vi "Pinholes.vi"(4 "Current Threshold [nA]":dbl, 5 "settling\ndelay":i32) -> (1 "excluded channels":i32[](array[numeric]), 2 "Current [nA]":dbl[](array[numeric]), 3 "Flag":i32[](array[numeric]))   [LabVIEW 2018]
uses:
  general_VIs/globals/QC_MeasurementSetup.vi
  InstrControl/Switching/Switching.lvclass
  InstrControl/SupplyControl/SupplyControl.lvclass
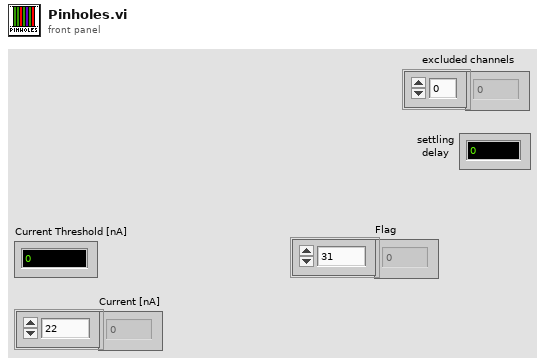
[diagram p1: front panel]
types:
  T1 = cluster{"Bias Supply":refnum<class "SupplyControl.lvclass">, "SMU":refnum<class "SupplyControl.lvclass">, "LCR":refnum<class "LCRControl.lvclass">, "ProbeStation":refnum<class "ProbeStationControl.lvclass">, "Arduino":refnum<class "ArduinoControl.lvclass">, "Measurement switch":refnum<class "Switching.lvclass">, "Probe Card Channels":i32, "Bias Voltage [V]":dbl, "First strip":i32, "Last strip":i32, "Base Voltage [V]":dbl, "Base Ramp Step [V]":dbl, "Base Ramp Interval [ms]":u32, "High Voltage [V]":dbl, "High Ramp Step [V]":dbl, "High Ramp Interval [ms]":u32, "AC frequency [Hz]":i32, "AC amplitude [V]":dbl, "RC Configuration":u16, "Single Needle":bool, "Temperature Readout":enum16{"Read Arduino", "Enter manually"}, "Fraction of good strips [%]":dbl, "Measurement switch used?":bool, "Matrix X Channels":cluster{"Mux1 C1":i32, "Mux1 C2":i32, "Mux2 C1":i32, "Mux2 C2":i32}, "Pinholes Y/N":bool, "Capacitance Y/N":bool, "Resistance Y/N":bool, "Bias Supply Name":string, "SMU Name":string, "LCR Name":string}
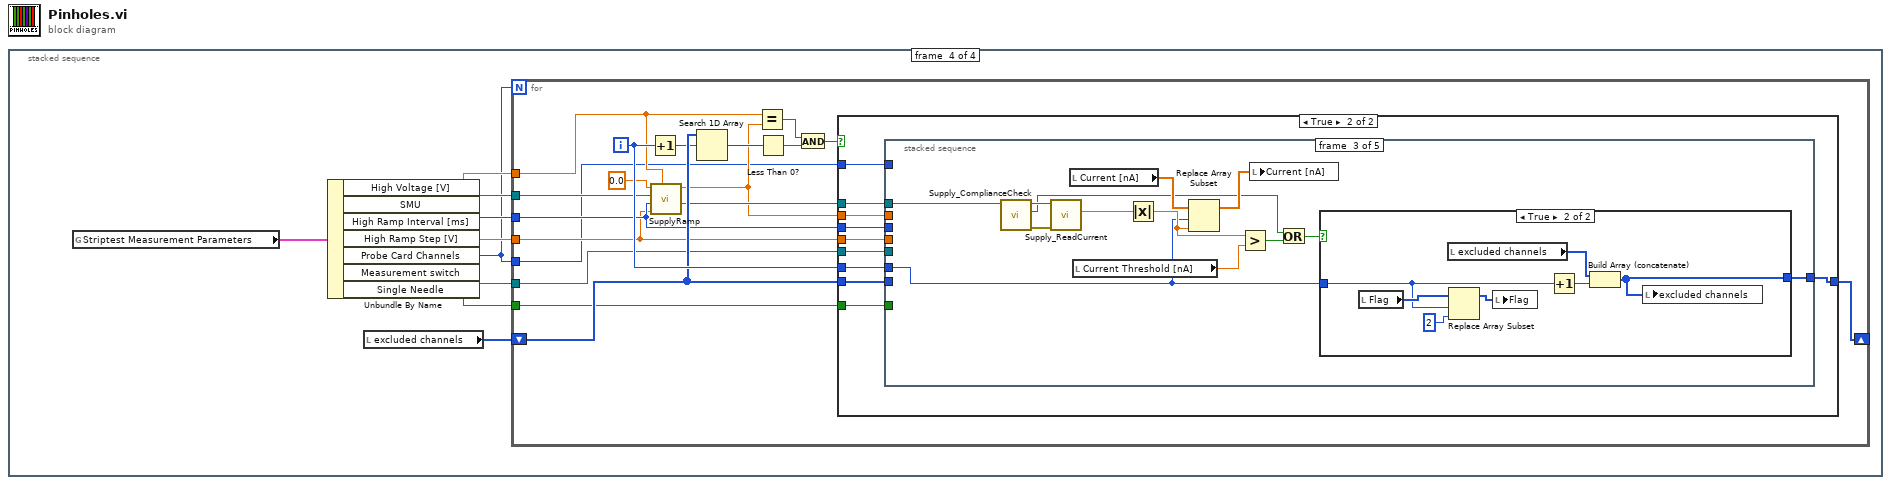
[diagram p0: block diagram]
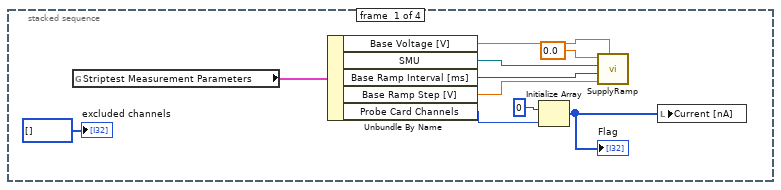
[diagram p2: hidden frame]
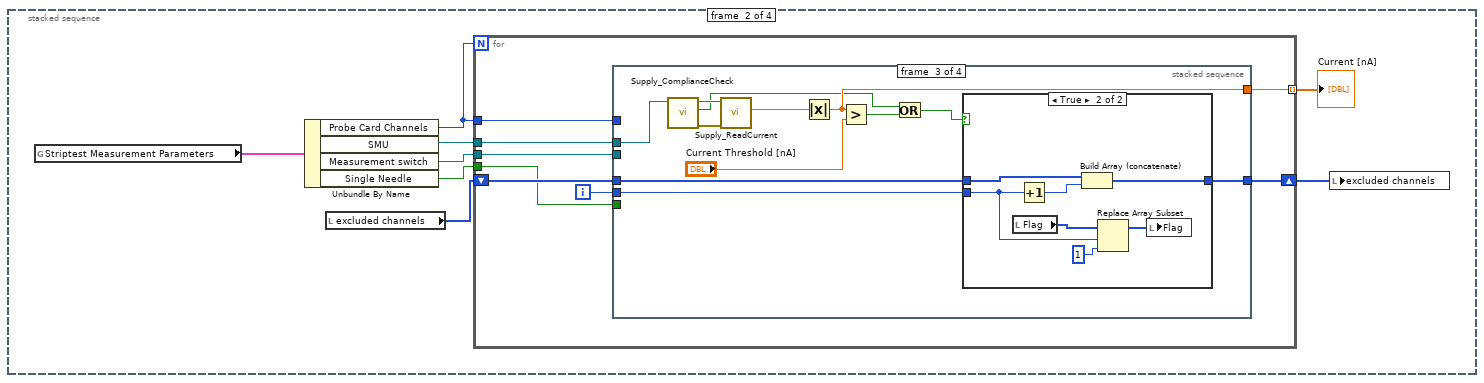
[diagram p3: hidden frame]
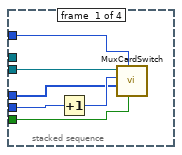
[diagram p4: hidden frame]
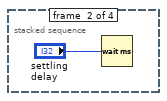
[diagram p5: hidden frame]
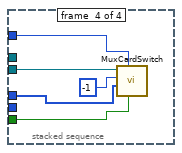
[diagram p7: hidden frame]
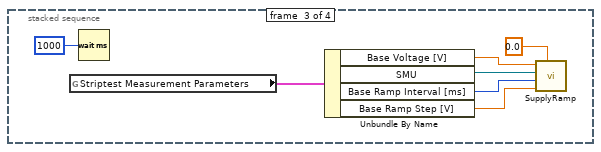
[diagram p8: hidden frame]
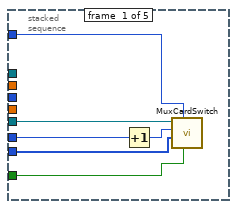
[diagram p10: hidden frame]
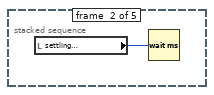
[diagram p11: hidden frame]
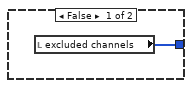
[diagram p12: hidden frame]
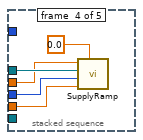
[diagram p13: hidden frame]
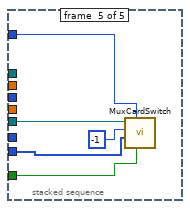
[diagram p14: hidden frame]
diagram:
  n1 = stacked-sequence {
    frame #0 {
      n2 = global read "QC_MeasurementSetup.vi" "Striptest Measurement Parameters"() -> (w6:T1)
      n3 = Unbundle By Name(w6) -> ("Base Voltage [V]"=w5:dbl, "SMU"=w1:refnum<class "SupplyControl.lvclass">, "Base Ramp Interval [ms]"=w4:u32, "Base Ramp Step [V]"=w3:dbl, "Probe Card Channels"=w2:i32)
      n4 = Initialize Array(0, w2) -> (w7:i32[])
      "Flag" <- w7
      n5 = call "SupplyRamp.vi"("Requested Voltage"=w5, "Step Size"=w3, "Step Delay"=w4, "Supply IN"=w1, "Starting Voltage"=0.0) -> ()  [unwired: 3 in, 4 out]
      n6 = local write "Current [nA]"(w7) -> ()
      "excluded channels" <- i32[] []
    }
    frame #1 {
      n7 = global read "QC_MeasurementSetup.vi" "Striptest Measurement Parameters"() -> (w16:T1)
      n8 = Unbundle By Name(w16) -> ("Probe Card Channels"=w11:i32, "SMU"=w15:refnum<class "SupplyControl.lvclass">, "Measurement switch"=w13:refnum<class "Switching.lvclass">, "Single Needle"=w12:bool)
      n9 = local read "excluded channels"() -> (w17:i32[])
      n10 = for {
        N: w11 -> [_]
        tunnel: w11 -> [w26]
        tunnel: [w25] -> w18 mode=indexing
        shift-right: [w22] -> w14
        shift-left: w17 -> [w24]
        tunnel: w13 -> [w19]
        tunnel: w12 -> [w21]
        tunnel: w15 -> [w20]
        i -> [w23]
        n11 = stacked-sequence {
          tunnel: w23 -> [w29 _ w34 _]
          tunnel: w26 -> [w31 _ _ w55]
          tunnel: w24 -> [w30 _ w36 w54]
          tunnel: [_ _ w41 _] -> w25
          tunnel: [_ _ w42 _] -> w22
          tunnel: w19 -> [w28 _ _ w57]
          tunnel: w21 -> [w27 _ _ w56]
          tunnel: w20 -> [_ _ w35 _]
          frame #0 {
            n12 = Increment(x=w29) -> (x+1=w32:i32)
            n13 = call-dynamic "MuxCardSwitch.vi"("Single Needle"=w27, "Probe Card Channels"=w31, "disabled channels"=w30, "Switch to channel"=w32, "Switching in"=w28) -> ()  [unwired: 4 in, 3 out]
          }
          frame #1 {
            n14 = Wait (ms)(milliseconds to wait="settling\ndelay") -> ()  [unwired: 1 out]
          }
          frame #2 {
            n15 = call-dynamic "Supply_ComplianceCheck.vi"("SupplyControl in"=w35) -> ("error out"=w40:errorcluster, "Compliance exceeded?"=w37:bool, "SupplyControl out"=w39:refnum<class "SupplyControl.lvclass">)  [unwired: 7 in, 1 out]
            n16 = call-dynamic "Supply_ReadCurrent.vi"("error in (no error)"=w40, "SupplyControl in"=w39) -> ("Current in nA"=w38:dbl)  [unwired: 7 in, 2 out]
            n17 = Absolute Value(x=w38) -> (abs(x)=w41:dbl)
            n18 = Greater?(x=w41, y="Current Threshold [nA]") -> (0:w43:bool)
            n19 = Or(x=w37, y=w43) -> (x .or. y?=w44:bool)
            n20 = case shown="True" w44 {
              tunnel: w36 -> [w46 w47]
              tunnel: [w46 w49] -> w42
              tunnel: w34 -> [_ w48]
              frame False {
              }
              frame True {
                n21 = local read "Flag"() -> (w53:i32[])
                n22 = Increment(x=w48) -> (x+1=w50:i32)
                n23 = Build Array (concatenate)(w47, w50) -> (w49:i32[])
                n24 = Replace Array Subset(array=w53, new element=1, index=w48) -> (w51:i32[])
                n25 = local write "Flag"(w51) -> ()
              }
            }
          }
          frame #3 {
            n26 = call-dynamic "MuxCardSwitch.vi"("Single Needle"=w56, "Probe Card Channels"=w55, "disabled channels"=w54, "Switch to channel"=-1, "Switching in"=w57) -> ()  [unwired: 4 in, 3 out]
          }
        }
      }
      "Current [nA]" <- w18
      n27 = local write "excluded channels"(w14) -> ()
    }
    frame #2 {
      n28 = global read "QC_MeasurementSetup.vi" "Striptest Measurement Parameters"() -> (w63:T1)
      n29 = Wait (ms)(milliseconds to wait=1000) -> ()  [unwired: 1 out]
      n30 = Unbundle By Name(w63) -> ("Base Voltage [V]"=w61:dbl, "SMU"=w62:refnum<class "SupplyControl.lvclass">, "Base Ramp Interval [ms]"=w60:u32, "Base Ramp Step [V]"=w59:dbl)
      n31 = call "SupplyRamp.vi"("Requested Voltage"=0.0, "Step Size"=w59, "Step Delay"=w60, "Supply IN"=w62, "Starting Voltage"=w61) -> ()  [unwired: 3 in, 4 out]
    }
    frame #3 {
      n32 = global read "QC_MeasurementSetup.vi" "Striptest Measurement Parameters"() -> (w73:T1)
      n33 = Unbundle By Name(w73) -> ("High Voltage [V]"=w72:dbl, "SMU"=w71:refnum<class "SupplyControl.lvclass">, "High Ramp Interval [ms]"=w70:u32, "High Ramp Step [V]"=w69:dbl, "Probe Card Channels"=w67:i32, "Measurement switch"=w68:refnum<class "Switching.lvclass">, "Single Needle"=w66:bool)
      n34 = local read "excluded channels"() -> (w74:i32[])
      n35 = for {
        N: w67 -> [_]
        shift-right: [w92] -> _
        shift-left: w74 -> [w90]
        tunnel: w72 -> [w81]
        tunnel: w71 -> [w80]
        tunnel: w70 -> [w79]
        tunnel: w69 -> [w78]
        tunnel: w68 -> [w77]
        tunnel: w67 -> [w76]
        tunnel: w66 -> [w75]
        i -> [w91]
        n36 = Increment(x=w91) -> (x+1=w89:i32)
        n37 = call "SupplyRamp.vi"("Requested Voltage"=w81, "Step Size"=w78, "Step Delay"=w79, "Supply IN"=w80, "Starting Voltage"=0.0) -> ("Supply OUT"=w83:refnum<class "SupplyControl.lvclass">, "Current Voltage"=w82:dbl)  [unwired: 3 in, 2 out]
        n38 = Search 1D Array(1D array=w90, element=w89) -> (index of element=w88:i32)  [unwired: 1 in]
        n39 = Equal?(x=w81, y=w82) -> (x = y?=w84:bool)
        n40 = Less Than 0?(x=w88) -> (x < 0?=w86:bool)
        n41 = And(x=w84, y=w86) -> (x .and. y?=w85:bool)
        n42 = case shown="True" w85 {
          tunnel: w90 -> [w93 w103]
          tunnel: w91 -> [_ w102]
          tunnel: [w93 w101] -> w92
          tunnel: w78 -> [_ w100]
          tunnel: w76 -> [_ w99]
          tunnel: w77 -> [_ w98]
          tunnel: w75 -> [_ w97]
          tunnel: w83 -> [_ w96]
          tunnel: w82 -> [_ w95]
          tunnel: w79 -> [_ w94]
          frame False {
          }
          frame True {
            n43 = stacked-sequence {
              tunnel: w102 -> [w107 _ w111 _ _]
              tunnel: w103 -> [w108 _ _ _ w137]
              tunnel: [_ _ w121 _ _] -> w101
              tunnel: w100 -> [_ _ _ w132 _]
              tunnel: w99 -> [w106 _ _ _ w138]
              tunnel: w98 -> [w105 _ _ _ w140]
              tunnel: w97 -> [w104 _ _ _ w139]
              tunnel: w96 -> [_ _ w113 w135 _]
              tunnel: w95 -> [_ _ _ w134 _]
              tunnel: w94 -> [_ _ _ w133 _]
              frame #0 {
                n44 = Increment(x=w107) -> (x+1=w109:i32)
                n45 = call-dynamic "MuxCardSwitch.vi"("Single Needle"=w104, "Probe Card Channels"=w106, "disabled channels"=w108, "Switch to channel"=w109, "Switching in"=w105) -> ()  [unwired: 4 in, 3 out]
              }
              frame #1 {
                n46 = local read "settling\ndelay"() -> (w110:i32)
                n47 = Wait (ms)(milliseconds to wait=w110) -> ()  [unwired: 1 out]
              }
              frame #2 {
                n48 = call-dynamic "Supply_ComplianceCheck.vi"("SupplyControl in"=w113) -> ("error out"=w115:errorcluster, "Compliance exceeded?"=w112:bool, "SupplyControl out"=w116:refnum<class "SupplyControl.lvclass">)  [unwired: 7 in, 1 out]
                n49 = call-dynamic "Supply_ReadCurrent.vi"("error in (no error)"=w115, "SupplyControl in"=w116) -> ("Current in nA"=w114:dbl)  [unwired: 7 in, 2 out]
                n50 = local read "Current [nA]"() -> (w118:dbl[])
                n51 = local read "Current Threshold [nA]"() -> (w120:dbl)
                n52 = Absolute Value(x=w114) -> (abs(x)=w117:dbl)
                n53 = Replace Array Subset(array=w118, new element=w117, index=w111) -> (w119:dbl[])
                n54 = Greater?(x=w117, y=w120) -> (0:w122:bool)
                n55 = local write "Current [nA]"(w119) -> ()
                n56 = Or(x=w112, y=w122) -> (x .or. y?=w123:bool)
                n57 = case shown="True" w123 {
                  tunnel: w111 -> [_ w127]
                  tunnel: [w124 w125] -> w121
                  frame False {
                    n58 = local read "excluded channels"() -> (w124:i32[])
                  }
                  frame True {
                    n59 = local read "Flag"() -> (w131:i32[])
                    n60 = local read "excluded channels"() -> (w128:i32[])
                    n61 = Replace Array Subset(array=w131, new element=2, index=w127) -> (w129:i32[])
                    n62 = local write "Flag"(w129) -> ()
                    n63 = Increment(x=w127) -> (x+1=w126:i32)
                    n64 = Build Array (concatenate)(w128, w126) -> (w125:i32[])
                    n65 = local write "excluded channels"(w125) -> ()
                  }
                }
              }
              frame #3 {
                n66 = call "SupplyRamp.vi"("Requested Voltage"=0.0, "Step Size"=w132, "Step Delay"=w133, "Supply IN"=w135, "Starting Voltage"=w134) -> ()  [unwired: 3 in, 4 out]
              }
              frame #4 {
                n67 = call-dynamic "MuxCardSwitch.vi"("Single Needle"=w139, "Probe Card Channels"=w138, "disabled channels"=w137, "Switch to channel"=-1, "Switching in"=w140) -> ()  [unwired: 4 in, 3 out]
              }
            }
          }
        }
      }
    }
  }
